vi "Single Calculate Limit Test Measurement Query.vi"(8 "error in":errorcluster, 10 "Calculation Channel":i32(ring) items=["Calc Channel 1", "Calc Channel 2", "Calc Channel 3", "Calc Channel 4"], 11 "Instrument Handle In":i32) -> (0 "error out":errorcluster, 2 "Measurement":i32(ring) items=["AC RMS", "Amplitude", "Average", "Cycle Average", "Cycle Frequency", "Cycle Period", "Cycle RMS", "DC RMS", "Effective Number of Bits", "Falling Edges", "Fall Overshoot", "Fall Preshoot", "Frequency", "Fall Crossing Time", "Fall Time", "High", "Low", "Maximum", "Minimum", "Mid", "Negative Duty", "Negative Width", "Positive Duty", "Period", "Phase", "Peak to Peak", "Pulse Width", "Rising Edges", "Rise Overshoot", "Rise Preshoot", "Rise Crossing Time", "Rise Time", "Standard Deviation", "Spurious Free Dynamic Range", "Spurious to Noise + Distortion", "Spurious to Noise", "Total Harmonic Distortion", "Time of Maximum", "Time of Minimum"], 3 "Instrument Handle Out":i32)   [LabVIEW 8.6, in "ZTScopeM.lvlib"]
doc: "Query which measurement is used for a limit test."
uses:
  ZTScopeM.lvlib
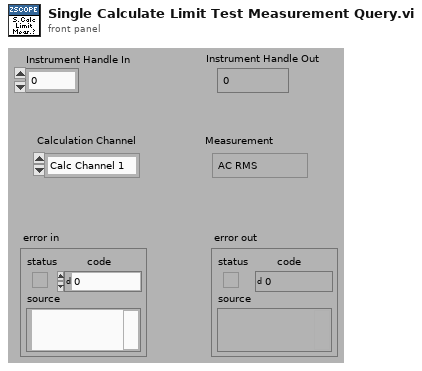
[diagram p1: front panel]
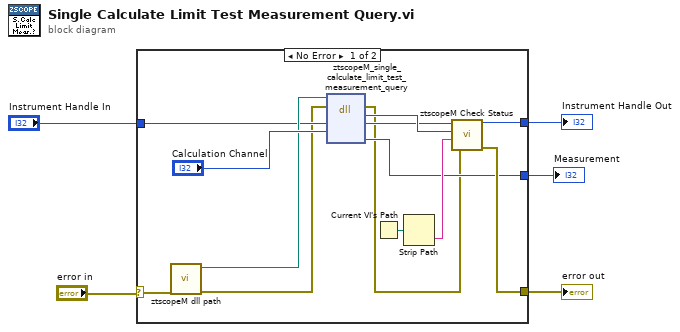
[diagram p0: block diagram]
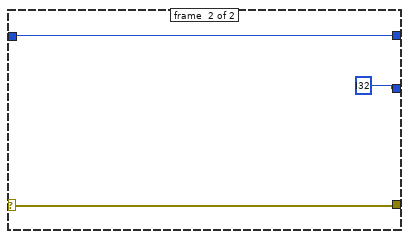
[diagram p2: hidden frame]
diagram:
  n1 = case shown="No Error" "error in" {
    selector: "error in" -> [w10 w21]
    tunnel: [w13 w21] -> w4
    tunnel: [w14 w19] -> w3
    tunnel: [w11 i32 ? ("instrumentHandle")] -> w2
    tunnel: "Instrument Handle In" -> [w8 w19]
    frame #0 {
      n2 = call "ztscopeM dll path.vi"("error in (no error)"=w10) -> ("error out"=w7:errorcluster, "<instrument>.dll path"=w9:path)  [unwired: 9 in]
      n3 = dll-call lib="C:/Program Files (x86)/National Instruments/LabVIEW 2013/instr.lib/ztscopem/ztscopeM.dll" fn="ztscopeM_single_calculate_limit_test_measurement_query"(path in=w9, error in=w7, "instrumentHandle"=w8, "calculationChannel"="Calculation Channel") -> (error out=w6:errorcluster, w18:i32, "instrumentHandle"=w17:i32, "measurement"=w11:i32)  [unwired: 2 in, 2 out]
      n4 = Current VI's Path() -> (path=w16:path)
      n5 = Strip Path(path=w16) -> (name=w15:string)  [unwired: 1 out]
      n6 = call "ztscopeM Check Status.vi"("error in"=w6, "name of VI"=w15, "status (return code)"=w18, "instrument handle in"=w17) -> ("error out"=w13:errorcluster, "instrument handle out"=w14:i32)  [unwired: 2 out]
    }
    frame #1 {
    }
  }
  "Instrument Handle Out" <- w3
  "error out" <- w4
  "Measurement" <- w2
